vi "move.vi"(8 "error in (no error)":errorcluster, 11 "Dog in":refnum<class "Dog.lvclass">) -> (0 "error out":errorcluster, 2 "message":string, 3 "Dog out":refnum<class "Dog.lvclass">)   [LabVIEW 2017, in "Dog.lvclass"]
uses:
  Dog.lvclass
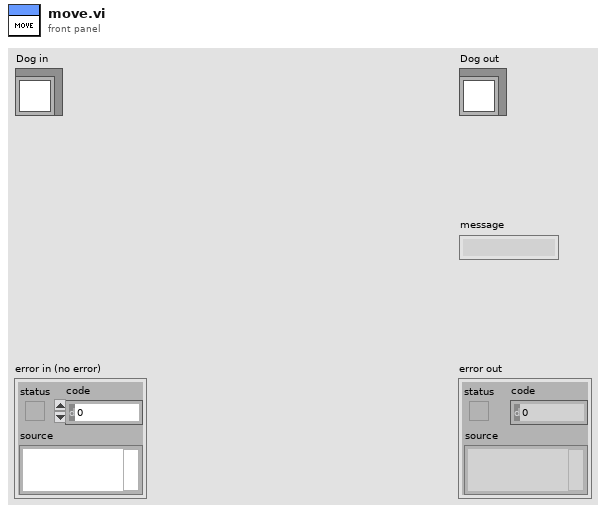
[diagram p1: front panel]
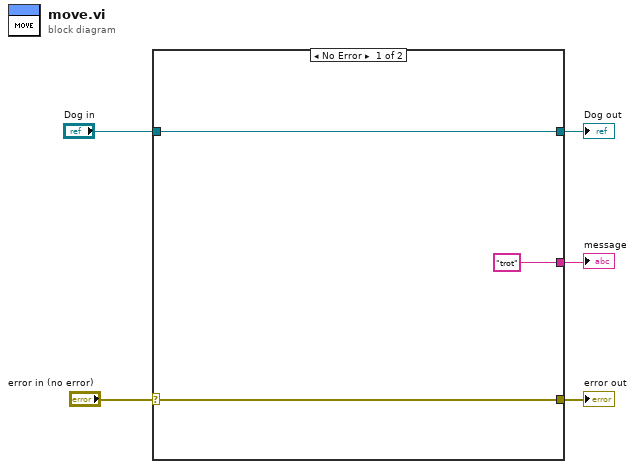
[diagram p0: block diagram]
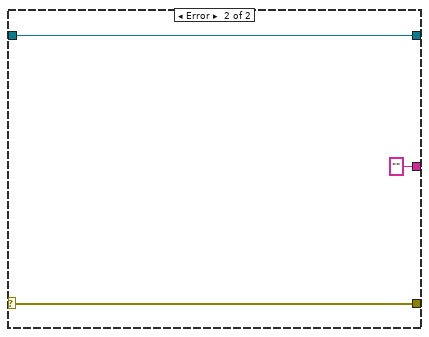
[diagram p2: hidden frame]
diagram:
  n1 = case shown="No Error" "error in (no error)" {
    selector: "error in (no error)" -> [w8 w9]
    tunnel: [w8 w9] -> w4
    tunnel: [w7 w11] -> w2
    tunnel: "Dog in" -> [w7 w11]
    tunnel: ["trot" ""] -> w1
    frame No Error {
    }
    frame Error {
    }
  }
  "error out" <- w4
  "Dog out" <- w2
  "message" <- w1
